vi "control rack tester.vi"() -> ()   [LabVIEW 2011]
panel:
  in  "stop":bool
  out "ai0 16":dynamicdata(graph) caption="data"
  out "ai0 15":dynamicdata(graph) caption="data"
  out "ai0 14":dynamicdata(graph) caption="data"
  out "ai0 13":dynamicdata(graph) caption="data"
  out "ai0 12":dynamicdata(graph) caption="data"
  out "ai0 11":dynamicdata(graph) caption="data"
  out "ai0 10":dynamicdata(graph) caption="data"
  out "ai0 9":dynamicdata(graph) caption="data"
  out "ai0 8":dynamicdata(graph) caption="data"
  out "ai0 7":dynamicdata(graph) caption="data"
  out "ai0 6":dynamicdata(graph) caption="data"
  out "ai0 5":dynamicdata(graph) caption="data"
  out "ai0 4":dynamicdata(graph) caption="data"
  out "ai0 3":dynamicdata(graph) caption="data"
  out "ai0 2":dynamicdata(graph) caption="data"
  out "ai0":dynamicdata(graph) caption="data"
  # "hel voltage feedback"
  # "voltage setpoint torr"
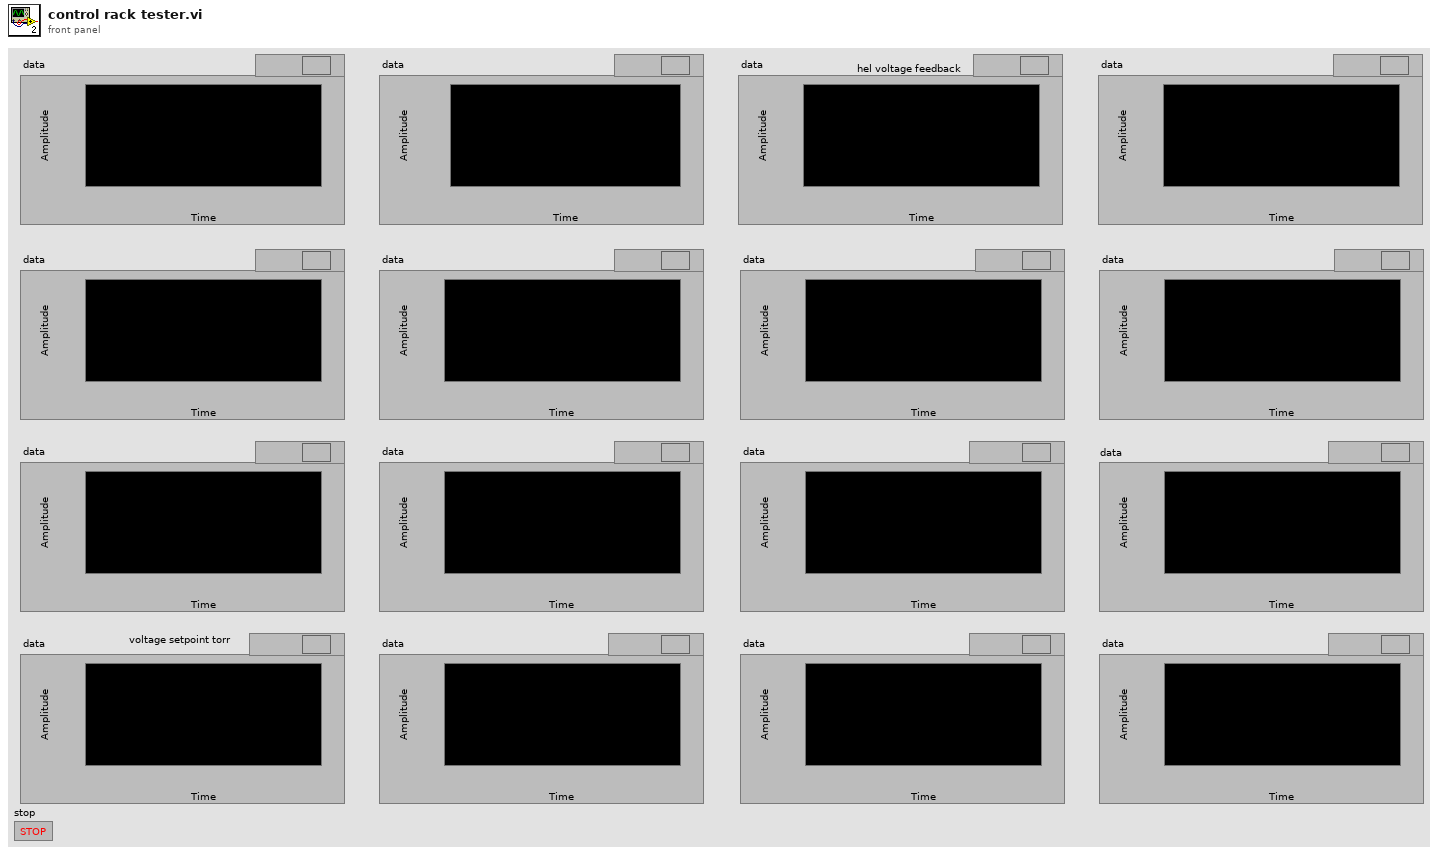
[diagram p1: front panel]
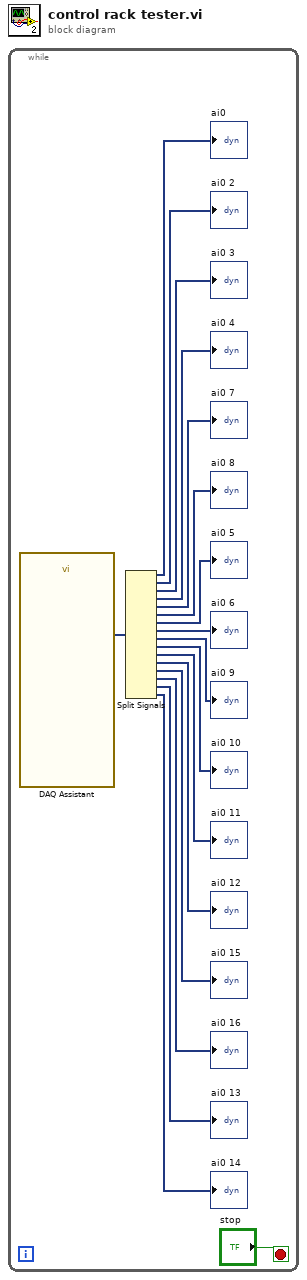
[diagram p0: block diagram]
diagram:
  n1 = while {
    stop <- "stop" stop-if-true
    n2 = call "DAQ Assistant"() -> ("data"=w17:dynamicdata)  [unwired: 17 in, 2 out]
    n3 = Split Signals(w17) -> (→"ai0":dynamicdata, →"ai0 2":dynamicdata, →"ai0 3":dynamicdata, →"ai0 4":dynamicdata, →"ai0 7":dynamicdata, →"ai0 8":dynamicdata, →"ai0 5":dynamicdata, →"ai0 6":dynamicdata, →"ai0 9":dynamicdata, →"ai0 10":dynamicdata, →"ai0 11":dynamicdata, →"ai0 12":dynamicdata, →"ai0 15":dynamicdata, →"ai0 16":dynamicdata, →"ai0 13":dynamicdata, →"ai0 14":dynamicdata)  [unwired: 16 in]
  }
